vi "Format CSV.vi"(8 "error in (no error)":errorcluster, 9 "delimiter":string=",", 10 "CSV File Input":path, 11 "Original CSV Format":enum16{"OGnE", "WAN-OGE"}(ring)) -> (0 "error out":errorcluster, 1 "Parcel Length":i32[](array[numeric]), 3 "All Terminal Data":T1[](array[typedef]))   [LabVIEW 2017] (continued)
23:18:22.733", "2011-05-24 23:18:22.767", "2011-05-24 23:18:22.800", "2011-05-24 23:18:22.833", "2011-05-24 23:18:22.867", "2011-05-24 23:18:22.900", "2011-05-24 23:18:22.933", "2011-05-24 23:18:22.967", "2011-05-24 23:18:23.000", "2011-05-24 23:18:23.033", "2011-05-24 23:18:23.067", "2011-05-24 23:18:23.100", "2011-05-24 23:18:23.133", "2011-05-24 23:18:23.167", "2011-05-24 23:18:23.200", "2011-05-24 23:18:23.233", "2011-05-24 23:18:23.267", "2011-05-24 23:18:23.300", "2011-05-24 23:18:23.333", "2011-05-24 23:18:23.367", "2011-05-24 23:18:23.400", "2011-05-24 23:18:23.433", "2011-05-24 23:18:23.467", "2011-05-24 23:18:23.500", "2011-05-24 23:18:23.533", "2011-05-24 23:18:23.567", "2011-05-24 23:18:23.600", "2011-05-24 23:18:23.633", "2011-05-24 23:18:23.667", "2011-05-24 23:18:23.700", "2011-05-24 23:18:23.733", "2011-05-24 23:18:23.767", "2011-05-24 23:18:23.800", "2011-05-24 23:18:23.833", "2011-05-24 23:18:23.867", "2011-05-24 23:18:23.900", "2011-05-24 23:18:23.933", "2011-05-24 23:18:23.967", "2011-05-24 23:18:24.000", "2011-05-24 23:18:24.033", "2011-05-24 23:18:24.067", "2011-05-24 23:18:24.100", "2011-05-24 23:18:24.133", "2011-05-24 23:18:24.167", "2011-05-24 23:18:24.200", "2011-05-24 23:18:24.233", "2011-05-24 23:18:24.267", "2011-05-24 23:18:24.300", "2011-05-24 23:18:24.333", "2011-05-24 23:18:24.367", "2011-05-24 23:18:24.400", "2011-05-24 23:18:24.433", "2011-05-24 23:18:24.467", "2011-05-24 23:18:24.500", "2011-05-24 23:18:24.533", "2011-05-24 23:18:24.567", "2011-05-24 23:18:24.600", "2011-05-24 23:18:24.633", "2011-05-24 23:18:24.667", "2011-05-24 23:18:24.700", "2011-05-24 23:18:24.733", "2011-05-24 23:18:24.767", "2011-05-24 23:18:24.800", "2011-05-24 23:18:24.833", "2011-05-24 23:18:24.867", "2011-05-24 23:18:24.900", "2011-05-24 23:18:24.933", "2011-05-24 23:18:24.967", "2011-05-24 23:18:25.000", "2011-05-24 23:18:25.033", "2011-05-24 23:18:25.067", "2011-05-24 23:18:25.100", "2011-05-24 23:18:25.133", "2011-05-24 23:18:25.167", "2011-05-24 23:18:25.200", "2011-05-24 23:18:25.233", "2011-05-24 23:18:25.267", "2011-05-24 23:18:25.300", "2011-05-24 23:18:25.333", "2011-05-24 23:18:25.367", "2011-05-24 23:18:25.400", "2011-05-24 23:18:25.433", "2011-05-24 23:18:25.467", "2011-05-24 23:18:25.500", "2011-05-24 23:18:25.533", "2011-05-24 23:18:25.567", "2011-05-24 23:18:25.600", "2011-05-24 23:18:25.633", "2011-05-24 23:18:25.667", "2011-05-24 23:18:25.700", "2011-05-24 23:18:25.733", "2011-05-24 23:18:25.767", "2011-05-24 23:18:25.800", "2011-05-24 23:18:25.833", "2011-05-24 23:18:25.867", "2011-05-24 23:18:25.900", "2011-05-24 23:18:25.933", "2011-05-24 23:18:25.967", "2011-05-24 23:18:26.000", "2011-05-24 23:18:26.033", "2011-05-24 23:18:26.067", "2011-05-24 23:18:26.100", "2011-05-24 23:18:26.133", "2011-05-24 23:18:26.167", "2011-05-24 23:18:26.200", "2011-05-24 23:18:26.233", "2011-05-24 23:18:26.267", "2011-05-24 23:18:26.300", "2011-05-24 23:18:26.333", "2011-05-24 23:18:26.367", "2011-05-24 23:18:26.400", "2011-05-24 23:18:26.433", "2011-05-24 23:18:26.467", "2011-05-24 23:18:26.500", "2011-05-24 23:18:26.533", "2011-05-24 23:18:26.567", "2011-05-24 23:18:26.600", "2011-05-24 23:18:26.633", "2011-05-24 23:18:26.667", "2011-05-24 23:18:26.700", "2011-05-24 23:18:26.733", "2011-05-24 23:18:26.767", "2011-05-24 23:18:26.800", "2011-05-24 23:18:26.833", "2011-05-24 23:18:26.867", "2011-05-24 23:18:26.900", "2011-05-24 23:18:26.933", "2011-05-24 23:18:26.967", "2011-05-24 23:18:27.000", "2011-05-24 23:18:27.033", "2011-05-24 23:18:27.067", "2011-05-24 23:18:27.100", "2011-05-24 23:18:27.133", "2011-05-24 23:18:27.167", "2011-05-24 23:18:27.200", "2011-05-24 23:18:27.233", "2011-05-24 23:18:27.267", "2011-05-24 23:18:27.300", "2011-05-24 23:18:27.333", "2011-05-24 23:18:27.367", "2011-05-24 23:18:27.400", "2011-05-24 23:18:27.433", "2011-05-24 23:18:27.467", "2011-05-24 23:18:27.500", "2011-05-24 23:18:27.533", "2011-05-24 23:18:27.567", "2011-05-24 23:18:27.600", "2011-05-24 23:18:27.633", "2011-05-24 23:18:27.667", "2011-05-24 23:18:27.700", "2011-05-24 23:18:27.733", "2011-05-24 23:18:27.767", "2011-05-24 23:18:27.800", "2011-05-24 23:18:27.833", "2011-05-24 23:18:27.867", "2011-05-24 23:18:27.900", "2011-05-24 23:18:27.933", "2011-05-24 23:18:27.967", "2011-05-24 23:18:28.000", "2011-05-24 23:18:28.033", "2011-05-24 23:18:28.067", "2011-05-24 23:18:28.100", "2011-05-24 23:18:28.133", "2011-05-24 23:18:28.167", "2011-05-24 23:18:28.200", "2011-05-24 23:18:28.233", "2011-05-24 23:18:28.267", "2011-05-24 23:18:28.300", "2011-05-24 23:18:28.333", "2011-05-24 23:18:28.367", "2011-05-24 23:18:28.400", "2011-05-24 23:18:28.433", "2011-05-24 23:18:28.467", "2011-05-24 23:18:28.500", "2011-05-24 23:18:28.533", "2011-05-24 23:18:28.567", "2011-05-24 23:18:28.600", "2011-05-24 23:18:28.633", "2011-05-24 23:18:28.667", "2011-05-24 23:18:28.700", "2011-05-24 23:18:28.733", "2011-05-24 23:18:28.767", "2011-05-24 23:18:28.800", "2011-05-24 23:18:28.833", "2011-05-24 23:18:28.867", "2011-05-24 23:18:28.900", "2011-05-24 23:18:28.933", "2011-05-24 23:18:28.967", "2011-05-24 23:18:29.000", "2011-05-24 23:18:29.033", "2011-05-24 23:18:29.067", "2011-05-24 23:18:29.100", "2011-05-24 23:18:29.133", "2011-05-24 23:18:29.167", "2011-05-24 23:18:29.200", "2011-05-24 23:18:29.233", "2011-05-24 23:18:29.267", "2011-05-24 23:18:29.300", "2011-05-24 23:18:29.333", "2011-05-24 23:18:29.367", "2011-05-24 23:18:29.400", "2011-05-24 23:18:29.433", "2011-05-24 23:18:29.467", "2011-05-24 23:18:29.500", "2011-05-24 23:18:29.533", "2011-05-24 23:18:29.567", "2011-05-24 23:18:29.600", "2011-05-24 23:18:29.633", "2011-05-24 23:18:29.667", "2011-05-24 23:18:29.700", "2011-05-24 23:18:29.733", "2011-05-24 23:18:29.767", "2011-05-24 23:18:29.800", "2011-05-24 23:18:29.833", "2011-05-24 23:18:29.867", "2011-05-24 23:18:29.900", "2011-05-24 23:18:29.933", "2011-05-24 23:18:29.967", "2011-05-24 23:18:30.000", "2011-05-24 23:18:30.033", "2011-05-24 23:18:30.067", "2011-05-24 23:18:30.100", "2011-05-24 23:18:30.133", "2011-05-24 23:18:30.167", "2011-05-24 23:18:30.200", "2011-05-24 23:18:30.233", "2011-05-24 23:18:30.267", "2011-05-24 23:18:30.300", "2011-05-24 23:18:30.333", "2011-05-24 23:18:30.367", "2011-05-24 23:18:30.400", "2011-05-24 23:18:30.433", "2011-05-24 23:18:30.467", "2011-05-24 23:18:30.500", "2011-05-24 23:18:30.533", "2011-05-24 23:18:30.567", "2011-05-24 23:18:30.600", "2011-05-24 23:18:30.633", "2011-05-24 23:18:30.667", "2011-05-24 23:18:30.700", "2011-05-24 23:18:30.733", "2011-05-24 23:18:30.767", "2011-05-24 23:18:30.800", "2011-05-24 23:18:30.833", "2011-05-24 23:18:30.867", "2011-05-24 23:18:30.900", "2011-05-24 23:18:30.933", "2011-05-24 23:18:30.967", "2011-05-24 23:18:31.000", "2011-05-24 23:18:31.033", "2011-05-24 23:18:31.067", "2011-05-24 23:18:31.100", "2011-05-24 23:18:31.133", "2011-05-24 23:18:31.167", "2011-05-24 23:18:31.200", "2011-05-24 23:18:31.233", "2011-05-24 23:18:31.267", "2011-05-24 23:18:31.300", "2011-05-24 23:18:31.333", "2011-05-24 23:18:31.367", "2011-05-24 23:18:31.400", "2011-05-24 23:18:31.433", "2011-05-24 23:18:31.467", "2011-05-24 23:18:31.500", "2011-05-24 23:18:31.533", "2011-05-24 23:18:31.567", "2011-05-24 23:18:31.600", "2011-05-24 23:18:31.633", "2011-05-24 23:18:31.667", "2011-05-24 23:18:31.700", "2011-05-24 23:18:31.733", "2011-05-24 23:18:31.767", "2011-05-24 23:18:31.800", "2011-05-24 23:18:31.833", "2011-05-24 23:18:31.867", "2011-05-24 23:18:31.900", "2011-05-24 23:18:31.933", "2011-05-24 23:18:31.967", "2011-05-24 23:18:32.000", "2011-05-24 23:18:32.033", "2011-05-24 23:18:32.067", "2011-05-24 23:18:32.100", "2011-05-24 23:18:32.133", "2011-05-24 23:18:32.167", "2011-05-24 23:18:32.200", "2011-05-24 23:18:32.233", "2011-05-24 23:18:32.267", "2011-05-24 23:18:32.300", "2011-05-24 23:18:32.333", "2011-05-24 23:18:32.367", "2011-05-24 23:18:32.400", "2011-05-24 23:18:32.433", "2011-05-24 23:18:32.467", "2011-05-24 23:18:32.500", "2011-05-24 23:18:32.533", "2011-05-24 23:18:32.567", "2011-05-24 23:18:32.600", "2011-05-24 23:18:32.633", "2011-05-24 23:18:32.667", "2011-05-24 23:18:32.700", "2011-05-24 23:18:32.733", "2011-05-24 23:18:32.767", "2011-05-24 23:18:32.800", "2011-05-24 23:18:32.833", "2011-05-24 23:18:32.867", "2011-05-24 23:18:32.900", "2011-05-24 23:18:32.933", "2011-05-24 23:18:32.967", "2011-05-24 23:18:33.000", "2011-05-24 23:18:33.033", "2011-05-24 23:18:33.067", "2011-05-24 23:18:33.100", "2011-05-24 23:18:33.133", "2011-05-24 23:18:33.167", "2011-05-24 23:18:33.200", "2011-05-24 23:18:33.233", "2011-05-24 23:18:33.267", "2011-05-24 23:18:33.300", "2011-05-24 23:18:33.333", "2011-05-24 23:18:33.367", "2011-05-24 23:18:33.400", "2011-05-24 23:18:33.433", "2011-05-24 23:18:33.467", "2011-05-24 23:18:33.500", "2011-05-24 23:18:33.533", "2011-05-24 23:18:33.567", "2011-05-24 23:18:33.600", "2011-05-24 23:18:33.633", "2011-05-24 23:18:33.667", "2011-05-24 23:18:33.700", "2011-05-24 23:18:33.733", "2011-05-24 23:18:33.767", "2011-05-24 23:18:33.800", "2011-05-24 23:18:33.833", "2011-05-24 23:18:33.867", "2011-05-24 23:18:33.900", "2011-05-24 23:18:33.933", "2011-05-24 23:18:33.967", "2011-05-24 23:18:34.000", "2011-05-24 23:18:34.033", "2011-05-24 23:18:34.067", "2011-05-24 23:18:34.100", "2011-05-24 23:18:34.133", "2011-05-24 23:18:34.167", "2011-05-24 23:18:34.200", "2011-05-24 23:18:34.233", "2011-05-24 23:18:34.267", "2011-05-24 23:18:34.300", "2011-05-24 23:18:34.333", "2011-05-24 23:18:34.367", "2011-05-24 23:18:34.400", "2011-05-24 23:18:34.433", "2011-05-24 23:18:34.467", "2011-05-24 23:18:34.500", "2011-05-24 23:18:34.533", "2011-05-24 23:18:34.567", "2011-05-24 23:18:34.600", "2011-05-24 23:18:34.633", "2011-05-24 23:18:34.667", "2011-05-24 23:18:34.700", "2011-05-24 23:18:34.733", "2011-05-24 23:18:34.767", "2011-05-24 23:18:34.800", "2011-05-24 23:18:34.833", "2011-05-24 23:18:34.867", "2011-05-24 23:18:34.900", "2011-05-24 23:18:34.933", "2011-05-24 23:18:34.967", "2011-05-24 23:18:35.000", "2011-05-24 23:18:35.033", "2011-05-24 23:18:35.067", "2011-05-24 23:18:35.100", "2011-05-24 23:18:35.133", "2011-05-24 23:18:35.167", "2011-05-24 23:18:35.200", "2011-05-24 23:18:35.233", "2011-05-24 23:18:35.267", "2011-05-24 23:18:35.300", "2011-05-24 23:18:35.333", "2011-05-24 23:18:35.367", "2011-05-24 23:18:35.400", "2011-05-24 23:18:35.433", "2011-05-24 23:18:35.467", "2011-05-24 23:18:35.500", "2011-05-24 23:18:35.533", "2011-05-24 23:18:35.567", "2011-05-24 23:18:35.600", "2011-05-24 23:18:35.633", "2011-05-24 23:18:35.667", "2011-05-24 23:18:35.700", "2011-05-24 23:18:35.733", "2011-05-24 23:18:35.767", "2011-05-24 23:18:35.800", "2011-05-24 23:18:35.833", "2011-05-24 23:18:35.867", "2011-05-24 23:18:35.900", "2011-05-24 23:18:35.933", "2011-05-24 23:18:35.967", "2011-05-24 23:18:36.000", "2011-05-24 23:18:36.033", "2011-05-24 23:18:36.067", "2011-05-24 23:18:36.100", "2011-05-24 23:18:36.133", "2011-05-24 23:18:36.167", "2011-05-24 23:18:36.200", "2011-05-24 23:18:36.233", "2011-05-24 23:18:36.267", "2011-05-24 23:18:36.300", "2011-05-24 23:18:36.333", "2011-05-24 23:18:36.367", "2011-05-24 23:18:36.400", "2011-05-24 23:18:36.433", "2011-05-24 23:18:36.467", "2011-05-24 23:18:36.500", "2011-05-24 23:18:36.533", "2011-05-24 23:18:36.567", "2011-05-24 23:18:36.600", "2011-05-24 23:18:36.633", "2011-05-24 23:18:36.667", "2011-05-24 23:18:36.700", "2011-05-24 23:18:36.733", "2011-05-24 23:18:36.767", "2011-05-24 23:18:36.800", "2011-05-24 23:18:36.833", "2011-05-24 23:18:36.867", "2011-05-24 23:18:36.900", "2011-05-24 23:18:36.933", "2011-05-24 23:18:36.967", "2011-05-24 23:18:37.000", "2011-05-24 23:18:37.033", "2011-05-24 23:18:37.067", "2011-05-24 23:18:37.100", "2011-05-24 23:18:37.133", "2011-05-24 23:18:37.167", "2011-05-24 23:18:37.200", "2011-05-24 23:18:37.233", "2011-05-24 23:18:37.267", "2011-05-24 23:18:37.300", "2011-05-24 23:18:37.333", "2011-05-24 23:18:37.367", "2011-05-24 23:18:37.400", "2011-05-24 23:18:37.433", "2011-05-24 23:18:37.467", "2011-05-24 23:18:37.500", "2011-05-24 23:18:37.533", "2011-05-24 23:18:37.567", "2011-05-24 23:18:37.600", "2011-05-24 23:18:37.633", "2011-05-24 23:18:37.667", "2011-05-24 23:18:37.700", "2011-05-24 23:18:37.733", "2011-05-24 23:18:37.767", "2011-05-24 23:18:37.800", "2011-05-24 23:18:37.833", "2011-05-24 23:18:37.867", "2011-05-24 23:18:37.900", "2011-05-24 23:18:37.933", "2011-05-24 23:18:37.967", "2011-05-24 23:18:38.000", "2011-05-24 23:18:38.033", "2011-05-24 23:18:38.067", "2011-05-24 23:18:38.100", "2011-05-24 23:18:38.133", "2011-05-24 23:18:38.167", "2011-05-24 23:18:38.200", "2011-05-24 23:18:38.233", "2011-05-24 23:18:38.267", "2011-05-24 23:18:38.300", "2011-05-24 23:18:38.333", "2011-05-24 23:18:38.367", "2011-05-24 23:18:38.400", "2011-05-24 23:18:38.433", "2011-05-24 23:18:38.467", "2011-05-24 23:18:38.500", "2011-05-24 23:18:38.533", "2011-05-24 23:18:38.567", "2011-05-24 23:18:38.600", "2011-05-24 23:18:38.633", "2011-05-24 23:18:38.667", "2011-05-24 23:18:38.700", "2011-05-24 23:18:38.733", "2011-05-24 23:18:38.767", "2011-05-24 23:18:38.800", "2011-05-24 23:18:38.833", "2011-05-24 23:18:38.867", "2011-05-24 23:18:38.900", "2011-05-24 23:18:38.933", "2011-05-24 23:18:38.967", "2011-05-24 23:18:39.000", "2011-05-24 23:18:39.033", "2011-05-24 23:18:39.067", "2011-05-24 23:18:39.100", "2011-05-24 23:18:39.133", "2011-05-24 23:18:39.167", "2011-05-24 23:18:39.200", "2011-05-24 23:18:39.233", "2011-05-24 23:18:39.267", "2011-05-24 23:18:39.300", "2011-05-24 23:18:39.333", "2011-05-24 23:18:39.367", "2011-05-24 23:18:39.400", "2011-05-24 23:18:39.433", "2011-05-24 23:18:39.467", "2011-05-24 23:18:39.500", "2011-05-24 23:18:39.533", "2011-05-24 23:18:39.567", "2011-05-24 23:18:39.600", "2011-05-24 23:18:39.633", "2011-05-24 23:18:39.667", "2011-05-24 23:18:39.700", "2011-05-24 23:18:39.733", "2011-05-24 23:18:39.767", "2011-05-24 23:18:39.800", "2011-05-24 23:18:39.833", "2011-05-24 23:18:39.867", "2011-05-24 23:18:39.900", "2011-05-24 23:18:39.933", "2011-05-24 23:18:39.967", "2011-05-24 23:18:40.000", "2011-05-24 23:18:40.033", "2011-05-24 23:18:40.067", "2011-05-24 23:18:40.100", "2011-05-24 23:18:40.133", "2011-05-24 23:18:40.167", "2011-05-24 23:18:40.200", "2011-05-24 23:18:40.233", "2011-05-24 23:18:40.267", "2011-05-24 23:18:40.300", "2011-05-24 23:18:40.333", "2011-05-24 23:18:40.367", "2011-05-24 23:18:40.400", "2011-05-24 23:18:40.433", "2011-05-24 23:18:40.467", "2011-05-24 23:18:40.500", "2011-05-24 23:18:40.533", "2011-05-24 23:18:40.567", "2011-05-24 23:18:40.600", "2011-05-24 23:18:40.633", "2011-05-24 23:18:40.667", "2011-05-24 23:18:40.700", "2011-05-24 23:18:40.733", "2011-05-24 23:18:40.767", "2011-05-24 23:18:40.800", "2011-05-24 23:18:40.833", "2011-05-24 23:18:40.867", "2011-05-24 23:18:40.900", "2011-05-24 23:18:40.933", "2011-05-24 23:18:40.967", "2011-05-24 23:18:41.000", "2011-05-24 23:18:41.033", "2011-05-24 23:18:41.067", "2011-05-24 23:18:41.100", "2011-05-24 23:18:41.133", "2011-05-24 23:18:41.167", "2011-05-24 23:18:41.200", "2011-05-24 23:18:41.233", "2011-05-24 23:18:41.267", "2011-05-24 23:18:41.300", "2011-05-24 23:18:41.333", "2011-05-24 23:18:41.367", "2011-05-24 23:18:41.400", "2011-05-24 23:18:41.433", "2011-05-24 23:18:41.467", "2011-05-24 23:18:41.500", "2011-05-24 23:18:41.533", "2011-05-24 23:18:41.567", "2011-05-24 23:18:41.600", "2011-05-24 23:18:41.633", "2011-05-24 23:18:41.667", "2011-05-24 23:18:41.700", "2011-05-24 23:18:41.733", "2011-05-24 23:18:41.767", "2011-05-24 23:18:41.800", "2011-05-24 23:18:41.833", "2011-05-24 23:18:41.867", "2011-05-24 23:18:41.900", "2011-05-24 23:18:41.933", "2011-05-24 23:18:41.967", "2011-05-24 23:18:42.000", "2011-05-24 23:18:42.033", "2011-05-24 23:18:42.067", "2011-05-24 23:18:42.100", "2011-05-24 23:18:42.133", "2011-05-24 23:18:42.167", "2011-05-24 23:18:42.200", "2011-05-24 23:18:42.233", "2011-05-24 23:18:42.267", "2011-05-24 23:18:42.300", "2011-05-24 23:18:42.333", "2011-05-24 23:18:42.367", "2011-05-24 23:18:42.400", "2011-05-24 23:18:42.433", "2011-05-24 23:18:42.467", "2011-05-24 23:18:42.500", "2011-05-24 23:18:42.533", "2011-05-24 23:18:42.567", "2011-05-24 23:18:42.600", "2011-05-24 23:18:42.633", "2011-05-24 23:18:42.667", "2011-05-24 23:18:42.700", "2011-05-24 23:18:42.733", "2011-05-24 23:18:42.767", "2011-05-24 23:18:42.800", "2011-05-24 23:18:42.833", "2011-05-24 23:18:42.867", "2011-05-24 23:18:42.900", "2011-05-24 23:18:42.933", "2011-05-24 23:18:42.967", "2011-05-24 23:18:43.000", "2011-05-24 23:18:43.033", "2011-05-24 23:18:43.067", "2011-05-24 23:18:43.100", "2011-05-24 23:18:43.133", "2011-05-24 23:18:43.167", "2011-05-24 23:18:43.200", "2011-05-24 23:18:43.233", "2011-05-24 23:18:43.267", "2011-05-24 23:18:43.300", "2011-05-24 23:18:43.333", "2011-05-24 23:18:43.367", "2011-05-24 23:18:43.400", "2011-05-24 23:18:43.433", "2011-05-24 23:18:43.467", "2011-05-24 23:18:43.500", "2011-05-24 23:18:43.533", "2011-05-24 23:18:43.567", "2011-05-24 23:18:43.600", "2011-05-24 23:18:43.633", "2011-05-24 23:18:43.667", "2011-05-24 23:18:43.700", "2011-05-24 23:18:43.733", "2011-05-24 23:18:43.767", "2011-05-24 23:18:43.800", "2011-05-24 23:18:43.833", "2011-05-24 23:18:43.867", "2011-05-24 23:18:43.900", "2011-05-24 23:18:43.933", "2011-05-24 23:18:43.967", "2011-05-24 23:18:44.000", "2011-05-24 23:18:44.033", "2011-05-24 23:18:44.067", "2011-05-24 23:18:44.100", "2011-05-24 23:18:44.133", "2011-05-24 23:18:44.167", "2011-05-24 23:18:44.200", "2011-05-24 23:18:44.233", "2011-05-24 23:18:44.267", "2011-05-24 23:18:44.300", "2011-05-24 23:18:44.333", "2011-05-24 23:18:44.367", "2011-05-24 23:18:44.400", "2011-05-24 23:18:44.433", "2011-05-24 23:18:44.467", "2011-05-24 23:18:44.500", "2011-05-24 23:18:44.533", "2011-05-24 23:18:44.567", "2011-05-24 23:18:44.600", "2011-05-24 23:18:44.633", "2011-05-24 23:18:44.667", "2011-05-24 23:18:44.700", "2011-05-24 23:18:44.733", "2011-05-24 23:18:44.767", "2011-05-24 23:18:44.800", "2011-05-24 23:18:44.833", "2011-05-24 23:18:44.867", "2011-05-24 23:18:44.900", "2011-05-24 23:18:44.933", "2011-05-24 23:18:44.967", "2011-05-24 23:18:45.000", "2011-05-24 23:18:45.033", "2011-05-24 23:18:45.067", "2011-05-24 23:18:45.100", "2011-05-24 23:18:45.133", "2011-05-24 23:18:45.167", "2011-05-24 23:18:45.200", "2011-05-24 23:18:45.233", "2011-05-24 23:18:45.267", "2011-05-24 23:18:45.300", "2011-05-24 23:18:45.333", "2011-05-24 23:18:45.367", "2011-05-24 23:18:45.400", "2011-05-24 23:18:45.433", "2011-05-24 23:18:45.467", "2011-05-24 23:18:45.500", "2011-05-24 23:18:45.533", "2011-05-24 23:18:45.567", "2011-05-24 23:18:45.600", "2011-05-24 23:18:45.633", "2011-05-24 23:18:45.667", "2011-05-24 23:18:45.700", "2011-05-24 23:18:45.733", "2011-05-24 23:18:45.767", "2011-05-24 23:18:45.800", "2011-05-24 23:18:45.833", "2011-05-24 23:18:45.867", "2011-05-24 23:18:45.900", "2011-05-24 23:18:45.933", "2011-05-24 23:18:45.967", "2011-05-24 23:18:46.000", "2011-05-24 23:18:46.033", "2011-05-24 23:18:46.067", "2011-05-24 23:18:46.100", "2011-05-24 23:18:46.133", "2011-05-24 23:18:46.167", "2011-05-24 23:18:46.200", "2011-05-24 23:18:46.233", "2011-05-24 23:18:46.267", "2011-05-24 23:18:46.300", "2011-05-24 23:18:46.333", "2011-05-24 23:18:46.367", "2011-05-24 23:18:46.400", "2011-05-24 23:18:46.433", "2011-05-24 23:18:46.467", "2011-05-24 23:18:46.500", "2011-05-24 23:18:46.533", "2011-05-24 23:18:46.567", "2011-05-24 23:18:46.600", "2011-05-24 23:18:46.633", "2011-05-24 23:18:46.667", "2011-05-24 23:18:46.700", "2011-05-24 23:18:46.733", "2011-05-24 23:18:46.767", "2011-05-24 23:18:46.800", "2011-05-24 23:18:46.833", "2011-05-24 23:18:46.867", "2011-05-24 23:18:46.900", "2011-05-24 23:18:46.933", "2011-05-24 23:18:46.967", "2011-05-24 23:18:47.000", "2011-05-24 23:18:47.033", "2011-05-24 23:18:47.067", "2011-05-24 23:18:47.100", "2011-05-24 23:18:47.133", "2011-05-24 23:18:47.167", "2011-05-24 23:18:47.200", "2011-05-24 23:18:47.233", "2011-05-24 23:18:47.267", "2011-05-24 23:18:47.300", "2011-05-24 23:18:47.333", "2011-05-24 23:18:47.367", "2011-05-24 23:18:47.400", "2011-05-24 23:18:47.433", "2011-05-24 23:18:47.467", "2011-05-24 23:18:47.500", "2011-05-24 23:18:47.533", "2011-05-24 23:18:47.567", "2011-05-24 23:18:47.600", "2011-05-24 23:18:47.633", "2011-05-24 23:18:47.667", "2011-05-24 23:18:47.700", "2011-05-24 23:18:47.733", "2011-05-24 23:18:47.767", "2011-05-24 23:18:47.800", "2011-05-24 23:18:47.833", "2011-05-24 23:18:47.867", "2011-05-24 23:18:47.900", "2011-05-24 23:18:47.933", "2011-05-24 23:18:47.967", "2011-05-24 23:18:48.000", "2011-05-24 23:18:48.033", "2011-05-24 23:18:48.067", "2011-05-24 23:18:48.100", "2011-05-24 23:18:48.133", "2011-05-24 23:18:48.167", "2011-05-24 23:18:48.200", "2011-05-24 23:18:48.233", "2011-05-24 23:18:48.267", "2011-05-24 23:18:48.300", "2011-05-24 23:18:48.333", "2011-05-24 23:18:48.367", "2011-05-24 23:18:48.400", "2011-05-24 23:18:48.433", "2011-05-24 23:18:48.467", "2011-05-24 23:18:48.500", "2011-05-24 23:18:48.533", "2011-05-24 23:18:48.567", "2011-05-24 23:18:48.600", "2011-05-24 23:18:48.633", "2011-05-24 23:18:48.667", "2011-05-24 23:18:48.700", "2011-05-24 23:18:48.733", "2011-05-24 23:18:48.767", "2011-05-24 23:18:48.800", "2011-05-24 23:18:48.833", "2011-05-24 23:18:48.867", "2011-05-24 23:18:48.900", "2011-05-24 23:18:48.933", "2011-05-24 23:18:48.967", "2011-05-24 23:18:49.000", "2011-05-24 23:18:49.033", "2011-05-24 23:18:49.067", "2011-05-24 23:18:49.100", "2011-05-24 23:18:49.133", "2011-05-24 23:18:49.167", "2011-05-24 23:18:49.200", "2011-05-24 23:18:49.233", "2011-05-24 23:18:49.267", "2011-05-24 23:18:49.300", "2011-05-24 23:18:49.333", "2011-05-24 23:18:49.367", "2011-05-24 23:18:49.400", "2011-05-24 23:18:49.433", "2011-05-24 23:18:49.467", "2011-05-24 23:18:49.500", "2011-05-24 23:18:49.533", "2011-05-24 23:18:49.567", "2011-05-24 23:18:49.600", "2011-05-24 23:18:49.633", "2011-05-24 23:18:49.667", "2011-05-24 23:18:49.700", "2011-05-24 23:18:49.733", "2011-05-24 23:18:49.767", "2011-05-24 23:18:49.800", "2011-05-24 23:18:49.833", "2011-05-24 23:18:49.867", "2011-05-24 23:18:49.900", "2011-05-24 23:18:49.933", "2011-05-24 23:18:49.967", "2011-05-24 23:18:50.000", "2011-05-24 23:18:50.033", "2011-05-24 23:18:50.067", "2011-05-24 23:18:50.100", "2011-05-24 23:18:50.133", "2011-05-24 23:18:50.167", "2011-05-24 23:18:50.200", "2011-05-24 23:18:50.233", "2011-05-24 23:18:50.267", "2011-05-24 23:18:50.300", "2011-05-24 23:18:50.333", "2011-05-24 23:18:50.367", "2011-05-24 23:18:50.400", "2011-05-24 23:18:50.433", "2011-05-24 23:18:50.467", "2011-05-24 23:18:50.500", "2011-05-24 23:18:50.533", "2011-05-24 23:18:50.567", "2011-05-24 23:18:50.600", "2011-05-24 23:18:50.633", "2011-05-24 23:18:50.667", "2011-05-24 23:18:50.700", "2011-05-24 23:18:50.733", "2011-05-24 23:18:50.767", "2011-05-24 23:18:50.800", "2011-05-24 23:18:50.833", "2011-05-24 23:18:50.867", "2011-05-24 23:18:50.900", "2011-05-24 23:18:50.933", "2011-05-24 23:18:50.967", "2011-05-24 23:18:51.000", "2011-05-24 23:18:51.033", "2011-05-24 23:18:51.067", "2011-05-24 23:18:51.100", "2011-05-24 23:18:51.133", "2011-05-24 23:18:51.167", "2011-05-24 23:18:51.200", "2011-05-24 23:18:51.233", "2011-05-24 23:18:51.267", "2011-05-24 23:18:51.300", "2011-05-24 23:18:51.333", "2011-05-24 23:18:51.367", "2011-05-24 23:18:51.400", "2011-05-24 23:18:51.433", "2011-05-24 23:18:51.467", "2011-05-24 23:18:51.500", "2011-05-24 23:18:51.533", "2011-05-24 23:18:51.567", "2011-05-24 23:18:51.600", "2011-05-24 23:18:51.633", "2011-05-24 23:18:51.667", "2011-05-24 23:18:51.700", "2011-05-24 23:18:51.733", "2011-05-24 23:18:51.767", "2011-05-24 23:18:51.800", "2011-05-24 23:18:51.833", "2011-05-24 23:18:51.867", "2011-05-24 23:18:51.900", "2011-05-24 23:18:51.933", "2011-05-24 23:18:51.967", "2011-05-24 23:18:52.000", "2011-05-24 23:18:52.033", "2011-05-24 23:18:52.067", "2011-05-24 23:18:52.100", "2011-05-24 23:18:52.133", "2011-05-24 23:18:52.167", "2011-05-24 23:18:52.200", "2011-05-24 23:18:52.233", "2011-05-24 23:18:52.267", "2011-05-24 23:18:52.300", "2011-05-24 23:18:52.333", "2011-05-24 23:18:52.367", "2011-05-24 23:18:52.400", "2011-05-24 23:18:52.433", "2011-05-24 23:18:52.467", "2011-05-24 23:18:52.500", "2011-05-24 23:18:52.533", "2011-05-24 23:18:52.567", "2011-05-24 23:18:52.600", "2011-05-24 23:18:52.633", "2011-05-24 23:18:52.667", "2011-05-24 23:18:52.700", "2011-05-24 23:18:52.733", "2011-05-24 23:18:52.767", "2011-05-24 23:18:52.800", "2011-05-24 23:18:52.833", "2011-05-24 23:18:52.867", "2011-05-24 23:18:52.900", "2011-05-24 23:18:52.933", "2011-05-24 23:18:52.967", "2011-05-24 23:18:53.000", "2011-05-24 23:18:53.033", "2011-05-24 23:18:53.067", "2011-05-24 23:18:53.100", "2011-05-24 23:18:53.133", "2011-05-24 23:18:53.167", "2011-05-24 23:18:53.200", "2011-05-24 23:18:53.233", "2011-05-24 23:18:53.267", "2011-05-24 23:18:53.300", "2011-05-24 23:18:53.333", "2011-05-24 23:18:53.367", "2011-05-24 23:18:53.400", "2011-05-24 23:18:53.433", "2011-05-24 23:18:53.467", "2011-05-24 23:18:53.500", "2011-05-24 23:18:53.533", "2011-05-24 23:18:53.567", "2011-05-24 23:18:53.600", "2011-05-24 23:18:53.633", "2011-05-24 23:18:53.667", "2011-05-24 23:18:53.700", "2011-05-24 23:18:53.733", "2011-05-24 23:18:53.767", "2011-05-24 23:18:53.800", "2011-05-24 23:18:53.833", "2011-05-24 23:18:53.867", "2011-05-24 23:18:53.900", "2011-05-24 23:18:53.933", "2011-05-24 23:18:53.967", "2011-05-24 23:18:54.000", "2011-05-24 23:18:54.033", "2011-05-24 23:18:54.067", "2011-05-24 23:18:54.100", "2011-05-24 23:18:54.133", "2011-05-24 23:18:54.167", "2011-05-24 23:18:54.200", "2011-05-24 23:18:54.233", "2011-05-24 23:18:54.267", "2011-05-24 23:18:54.300", "2011-05-24 23:18:54.333", "2011-05-24 23:18:54.367", "2011-05-24 23:18:54.400", "2011-05-24 23:18:54.433", "2011-05-24 23:18:54.467", "2011-05-24 23:18:54.500", "2011-05-24 23:18:54.533", "2011-05-24 23:18:54.567", "2011-05-24 23:18:54.600", "2011-05-24 23:18:54.633", "2011-05-24 23:18:54.667", "2011-05-24 23:18:54.700", "2011-05-24 23:18:54.733", "2011-05-24 23:18:54.767", "2011-05-24 23:18:54.800", "2011-05-24 23:18:54.833", "2011-05-24 23:18:54.867", "2011-05-24 23:18:54.900", "2011-05-24 23:18:54.933", "2011-05-24 23:18:54.967", "2011-05-24 23:18:55.000", "2011-05-24 23:18:55.033", "2011-05-24 23:18:55.067", "2011-05-24 23:18:55.100", "2011-05-24 23:18:55.133", "2011-05-24 23:18:55.167", "2011-05-24 23:18:55.200", "2011-05-24 23:18:55.233", "2011-05-24 23:18:55.267", "2011-05-24 23:18:55.300", "2011-05-24 23:18:55.333", "2011-05-24 23:18:55.367", "2011-05-24 23:18:55.400", "2011-05-24 23:18:55.433", "2011-05-24 23:18:55.467", "2011-05-24 23:18:55.500", "2011-05-24 23:18:55.533", "2011-05-24 23:18:55.567", "2011-05-24 23:18:55.600", "2011-05-24 23:18:55.633", "2011-05-24 23:18:55.667", "2011-05-24 23:18:55.700", "2011-05-24 23:18:55.733", "2011-05-24 23:18:55.767", "2011-05-24 23:18:55.800", "2011-05-24 23:18:55.833", "2011-05-24 23:18:55.867", "2011-05-24 23:18:55.900", "2011-05-24 23:18:55.933", "2011-05-24 23:18:55.967", "2011-05-24 23:18:56.000", "2011-05-24 23:18:56.033", "2011-05-24 23:18:56.067", "2011-05-24 23:18:56.100", "2011-05-24 23:18:56.133", "2011-05-24 23:18:56.167", "2011-05-24 23:18:56.200", "2011-05-24 23:18:56.233", "2011-05-24 23:18:56.267", "2011-05-24 23:18:56.300", "2011-05-24 23:18:56.333", "2011-05-24 23:18:56.367", "2011-05-24 23:18:56.400", "2011-05-24 23:18:56.433", "2011-05-24 23:18:56.467", "2011-05-24 23:18:56.500", "2011-05-24 23:18:56.533", "2011-05-24 23:18:56.567", "2011-05-24 23:18:56.600", "2011-05-24 23:18:56.633", "2011-05-24 23:18:56.667", "2011-05-24 23:18:56.700", "2011-05-24 23:18:56.733", "2011-05-24 23:18:56.767", "2011-05-24 23:18:56.800", "2011-05-24 23:18:56.833", "2011-05-24 23:18:56.867", "2011-05-24 23:18:56.900", "2011-05-24 23:18:56.933", "2011-05-24 23:18:56.967", "2011-05-24 23:18:57.000", "2011-05-24 23:18:57.033", "2011-05-24 23:18:57.067", "2011-05-24 23:18:57.100", "2011-05-24 23:18:57.133", "2011-05-24 23:18:57.167", "2011-05-24 23:18:57.200", "2011-05-24 23:18:57.233", "2011-05-24 23:18:57.267", "2011-05-24 23:18:57.300", "2011-05-24 23:18:57.333", "2011-05-24 23:18:57.367", "2011-05-24 23:18:57.400", "2011-05-24 23:18:57.433", "2011-05-24 23:18:57.467", "2011-05-24 23:18:57.500", "2011-05-24 23:18:57.533", "2011-05-24 23:18:57.567", "2011-05-24 23:18:57.600", "2011-05-24 23:18:57.633", "2011-05-24 23:18:57.667", "2011-05-24 23:18:57.700", "2011-05-24 23:18:57.733", "2011-05-24 23:18:57.767", "2011-05-24 23:18:57.800", "2011-05-24 23:18:57.833", "2011-05-24 23:18:57.867", "2011-05-24 23:18:57.900", "2011-05-24 23:18:57.933", "2011-05-24 23:18:57.967", "2011-05-24 23:18:58.000", "2011-05-24 23:18:58.033", "2011-05-24 23:18:58.067", "2011-05-24 23:18:58.100", "2011-05-24 23:18:58.133", "2011-05-24 23:18:58.167", "2011-05-24 23:18:58.200", "2011-05-24 23:18:58.233", "2011-05-24 23:18:58.267", "2011-05-24 23:18:58.300", "2011-05-24 23:18:58.333", "2011-05-24 23:18:58.367", "2011-05-24 23:18:58.400", "2011-05-24 23:18:58.433", "2011-05-24 23:18:58.467", "2011-05-24 23:18:58.500", "2011-05-24 23:18:58.533", "2011-05-24 23:18:58.567", "2011-05-24 23:18:58.600", "2011-05-24 23:18:58.633", "2011-05-24 23:18:58.667", "2011-05-24 23:18:58.700", "2011-05-24 23:18:58.733", "2011-05-24 23:18:58.767", "2011-05-24 23:18:58.800", "2011-05-24 23:18:58.833", "2011-05-24 23:18:58.867", "2011-05-24 23:18:58.900", "2011-05-24 23:18:58.933", "2011-05-24 23:18:58.967", "2011-05-24 23:18:59.000", "2011-05-24 23:18:59.033", "2011-05-24 23:18:59.067", "2011-05-24 23:18:59.100", "2011-05-24 23:18:59.133", "2011-05-24 23:18:59.167", "2011-05-24 23:18:59.200", "2011-05-24 23:18:59.233", "2011-05-24 23:18:59.267", "2011-05-24 23:18:59.300", "2011-05-24 23:18:59.333", "2011-05-24 23:18:59.367", "2011-05-24 23:18:59.400", "2011-05-24 23:18:59.433", "2011-05-24 23:18:59.467", "2011-05-24 23:18:59.500", "2011-05-24 23:18:59.533", "2011-05-24 23:18:59.567", "2011-05-24 23:18:59.600", "2011-05-24 23:18:59.633", "2011-05-24 23:18:59.667", "2011-05-24 23:18:59.700", "2011-05-24 23:18:59.733", "2011-05-24 23:18:59.767", "2011-05-24 23:18:59.800", "2011-05-24 23:18:59.833", "2011-05-24 23:18:59.867", "2011-05-24 23:18:59.900", "2011-05-24 23:18:59.933", "2011-05-24 23:18:59.967", "2011-05-24 23:19:00.000", "2011-05-24 23:19:00.033", "2011-05-24 23:19:00.067", "2011-05-24 23:19:00.100", "2011-05-24 23:19:00.133", "2011-05-24 23:19:00.167", "2011-05-24 23:19:00.200", "2011-05-24 23:19:00.233", "2011-05-24 23:19:00.267", "2011-05-24 23:19:00.300", "2011-05-24 23:19:00.333", "2011-05-24 23:19:00.367", "2011-05-24 23:19:00.400", "2011-05-24 23:19:00.433", "2011-05-24 23:19:00.467", "2011-05-24 23:19:00.500", "2011-05-24 23:19:00.533", "2011-05-24 23:19:00.567", "2011-05-24 23:19:00.600", "2011-05-24 23:19:00.633", "2011-05-24 23:19:00.667", "2011-05-24 23:19:00.700", "2011-05-24 23:19:00.733", "2011-05-24 23:19:00.767", "2011-05-24 23:19:00.800", "2011-05-24 23:19:00.833", "2011-05-24 23:19:00.867", "2011-05-24 23:19:00.900", "2011-05-24 23:19:00.933", "2011-05-24 23:19:00.967", "2011-05-24 23:19:01.000", "2011-05-24 23:19:01.033", "2011-05-24 23:19:01.067", "2011-05-24 23:19:01.100", "2011-05-24 23:19:01.133", "2011-05-24 23:19:01.167", "2011-05-24 23:19:01.200", "2011-05-24 23:19:01.233", "2011-05-24 23:19:01.267", "2011-05-24 23:19:01.300", "2011-05-24 23:19:01.333", "2011-05-24 23:19:01.367", "2011-05-24 23:19:01.400", "2011-05-24 23:19:01.433", "2011-05-24 23:19:01.467", "2011-05-24 23:19:01.500", "2011-05-24 23:19:01.533", "2011-05-24 23:19:01.567", "2011-05-24 23:19:01.600", "2011-05-24 23:19:01.633", "2011-05-24 23:19:01.667", "2011-05-24 23:19:01.700", "2011-05-24 23:19:01.733", "2011-05-24 23:19:01.767", "2011-05-24 23:19:01.800", "2011-05-24 23:19:01.833", "2011-05-24 23:19:01.867", "2011-05-24 23:19:01.900", "2011-05-24 23:19:01.933", "2011-05-24 23:19:01.967", "2011-05-24 23:19:02.000", "2011-05-24 23:19:02.033", "2011-05-24 23:19:02.067", "2011-05-24 23:19:02.100", "2011-05-24 23:19:02.133", "2011-05-24 23:19:02.167", "2011-05-24 23:19:02.200", "2011-05-24 23:19:02.233", "2011-05-24 23:19:02.267", "2011-05-24 23:19:02.300", "2011-05-24 23:19:02.333", "2011-05-24 23:19:02.367", "2011-05-24 23:19:02.400", "2011-05-24 23:19:02.433", "2011-05-24 23:19:02.467", "2011-05-24 23:19:02.500", "2011-05-24 23:19:02.533", "2011-05-24 23:19:02.567", "2011-05-24 23:19:02.600", "2011-05-24 23:19:02.633", "2011-05-24 23:19:02.667", "2011-05-24 23:19:02.700", "2011-05-24 23:19:02.733", "2011-05-24 23:19:02.767", "2011-05-24 23:19:02.800", "2011-05-24 23:19:02.833", "2011-05-24 23:19:02.867", "2011-05-24 23:19:02.900", "2011-05-24 23:19:02.933", "2011-05-24 23:19:02.967", "2011-05-24 23:19:03.000", "2011-05-24 23:19:03.033", "2011-05-24 23:19:03.067", "2011-05-24 23:19:03.100", "2011-05-24 23:19:03.133", "2011-05-24 23:19:03.167", "2011-05-24 23:19:03.200", "2011-05-24 23:19:03.233", "2011-05-24 23:19:03.267", "2011-05-24 23:19:03.300", "2011-05-24 23:19:03.333", "2011-05-24 23:19:03.367", "2011-05-24 23:19:03.400", "2011-05-24 23:19:03.433", "2011-05-24 23:19:03.467", "2011-05-24 23:19:03.500", "2011-05-24 23:19:03.533", "2011-05-24 23:19:03.567", "2011-05-24 23:19:03.600", "2011-05-24 23:19:03.633", "2011-05-24 23:19:03.667", "2011-05-24 23:19:03.700", "2011-05-24 23:19:03.733", "2011-05-24 23:19:03.767", "2011-05-24 23:19:03.800", "2011-05-24 23:19:03.833", "2011-05-24 23:19:03.867", "2011-05-24 23:19:03.900", "2011-05-24 23:19:03.933", "2011-05-24 23:19:03.967", "2011-05-24 23:19:04.000", "2011-05-24 23:19:04.033", "2011-05-24 23:19:04.067", "2011-05-24 23:19:04.100", "2011-05-24 23:19:04.133", "2011-05-24 23:19:04.167", "2011-05-24 23:19:04.200", "2011-05-24 23:19:04.233", "2011-05-24 23:19:04.267", "2011-05-24 23:19:04.300", "2011-05-24 23:19:04.333", "2011-05-24 23:19:04.367", "2011-05-24 23:19:04.400", "2011-05-24 23:19:04.433", "2011-05-24 23:19:04.467", "2011-05-24 23:19:04.500", "2011-05-24 23:19:04.533", "2011-05-24 23:19:04.567", "2011-05-24 23:19:04.600", "2011-05-24 23:19:04.633", "2011-05-24 23:19:04.667", "2011-05-24 23:19:04.700", "2011-05-24 23:19:04.733", "2011-05-24 23:19:04.767", "2011-05-24 23:19:04.800", "2011-05-24 23:19:04.833", "2011-05-24 23:19:04.867", "2011-05-24 23:19:04.900", "2011-05-24 23:19:04.933", "2011-05-24 23:19:04.967", "2011-05-24 23:19:05.000", "2011-05-24 23:19:05.033", "2011-05-24 23:19:05.067", "2011-05-24 23:19:05.100", "2011-05-24 23:19:05.133", "2011-05-24 23:19:05.167", "2011-05-24 23:19:05.200", "2011-05-24 23:19:05.233", "2011-05-24 23:19:05.267", "2011-05-24 23:19:05.300", "2011-05-24 23:19:05.333", "2011-05-24 23:19:05.367", "2011-05-24 23:19:05.400", "2011-05-24 23:19:05.433", "2011-05-24 23:19:05.467", "2011-05-24 23:19:05.500", "2011-05-24 23:19:05.533", "2011-05-24 23:19:05.567", "2011-05-24 23:19:05.600", "2011-05-24 23:19:05.633", "2011-05-24 23:19:05.667", "2011-05-24 23:19:05.700", "2011-05-24 23:19:05.733", "2011-05-24 23:19:05.767", "2011-05-24 23:19:05.800", "2011-05-24 23:19:05.833", "2011-05-24 23:19:05.867", "2011-05-24 23:19:05.900"]
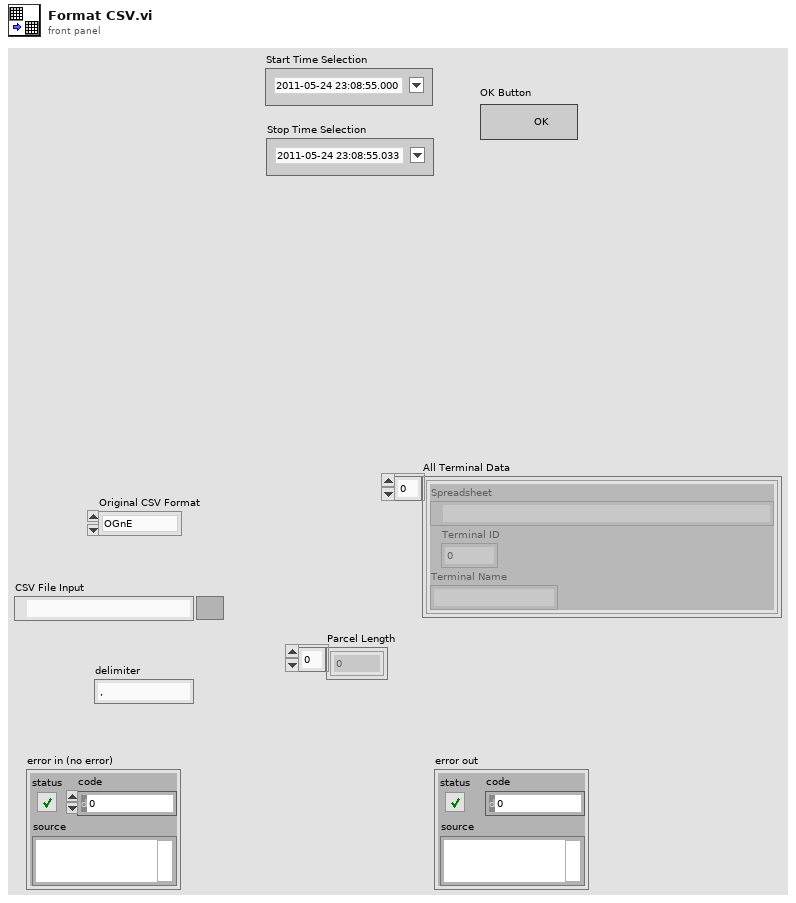
[diagram p1: front panel]
types:
  T1 = typedef "Terminal Data.ctl" = cluster{"Spreadsheet":path, "Terminal ID":u32, "Terminal Name":string}
  T2 = enum8{"Enabled", "Disabled", "Disabled and Grayed Out"}
  T3 = cluster{"Terminal Data":path, "Terminal ID":dbl, "Terminal Name":string}
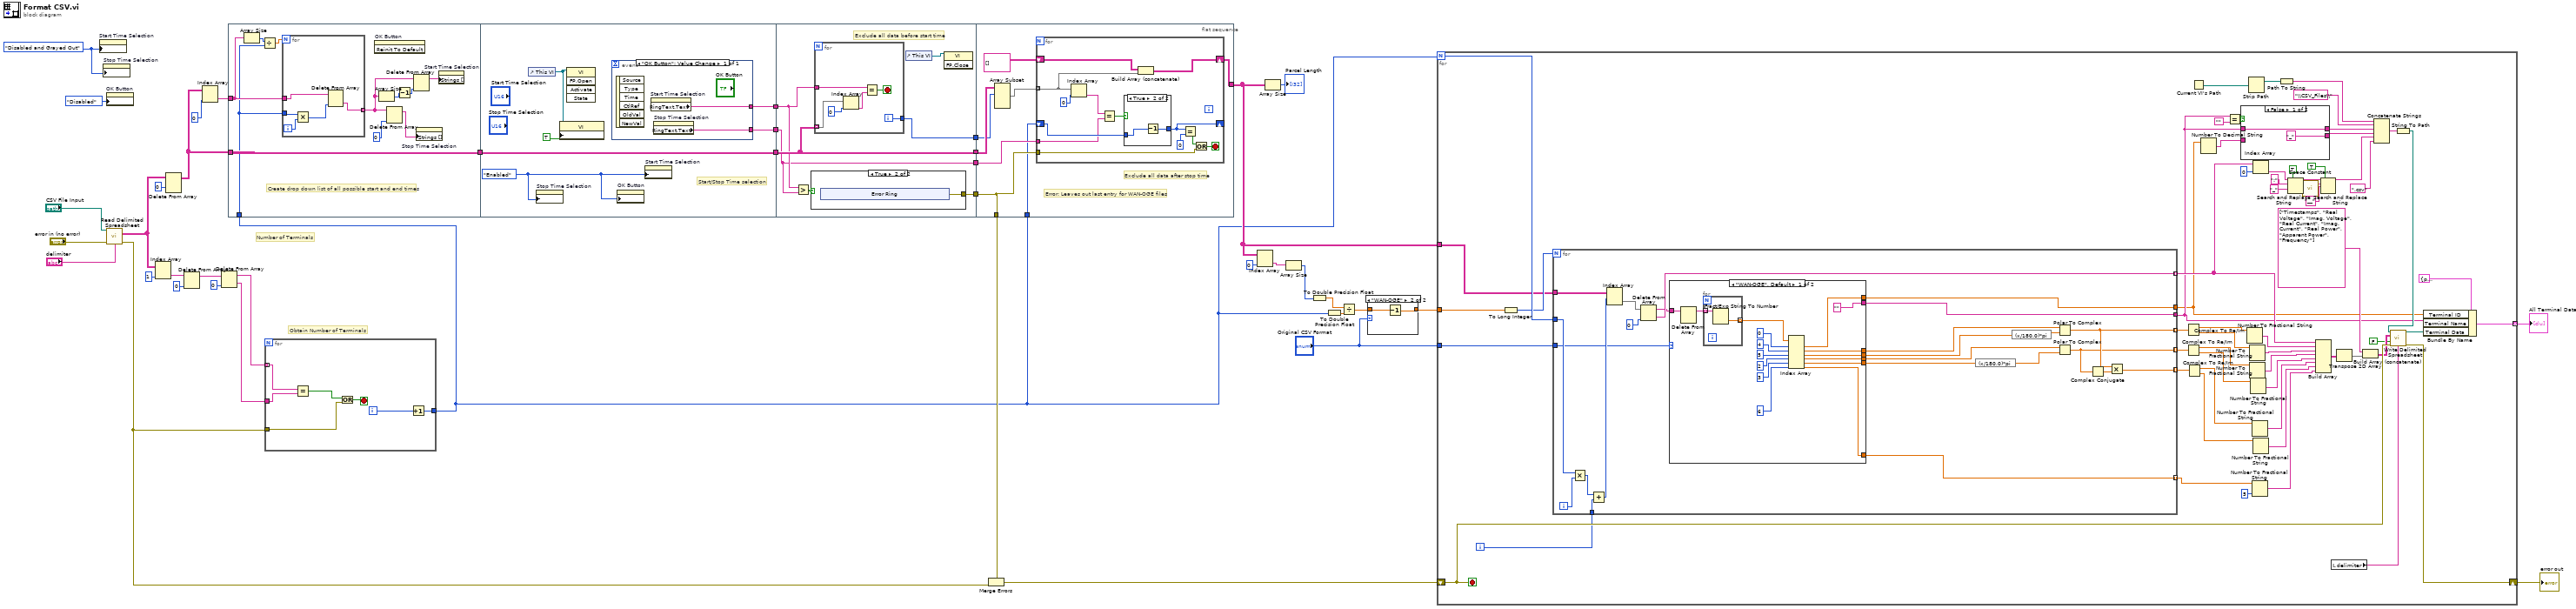
[diagram p0: block diagram]
diagram:
  w2 = T2."Disabled and Grayed Out" ("Disabled")
  # "Obtain Number of Terminals"
  # "Number of Terminals"
  n1 = property on="Start Time Selection" class="Ring (strict)"("DisabledEnum"=w2) -> ()  [unwired: 2 in, 2 out]
  n2 = property on="Stop Time Selection" class="Ring (strict)"("DisabledEnum"=w2) -> ()  [unwired: 2 in, 2 out]
  n3 = property on="OK Button" class="Bool"("DisabledEnum"=T2."Disabled" ("Disabled")) -> ()  [unwired: 2 in, 2 out]
  n4 = call-poly <vilib>:"Read Delimited Spreadsheet.vi"("file path (dialog if empty)"="CSV File Input", "error in (no error)"="error in (no error)", "delimiter (\\t)"="delimiter") -> ("all rows"=w21:string[][], "error out"=w12:errorcluster)  [unwired: 7 in, 4 out]
  n5 = Index Array(array=w21, index (col)=1 ("disabled index (col)")) -> (element=w27:string[])  [unwired: 1 in]
  n6 = Delete From Array(array=w21, index (row)=0) -> (array with subset deleted=w19:string[][])  [unwired: 2 in, 1 out]
  n7 = Delete From Array(array=w27, index=0) -> (array with subset deleted=w26:string[])  [unwired: 1 in, 1 out]
  n8 = Index Array(array=w19, index (col)=0 ("disabled index (col)")) -> (element=w22:string[])  [unwired: 1 in]
  n9 = Delete From Array(array=w26, index=0) -> (deleted portion=w35:string, array with subset deleted=w36:string[])  [unwired: 1 in]
  n10 = flat-sequence {
    tunnel: [w52] -> w24
    tunnel: w19 -> [w52]
    tunnel: w22 -> [w51]
    tunnel: w3 -> [w46]
    tunnel: w24 -> [w63]
    tunnel: [w63] -> w18
    tunnel: [w60] -> w17
    tunnel: [w59] -> w16
    tunnel: w18 -> [w72]
    tunnel: w17 -> [w70]
    tunnel: w16 -> [w69]
    tunnel: [w69] -> w15
    tunnel: [w72] -> w14
    tunnel: [w71] -> w13
    tunnel: [w67] -> w10
    tunnel: [w94] -> w5
    tunnel: w15 -> [w91]
    tunnel: w14 -> [w92]
    tunnel: w13 -> [w90]
    tunnel: w3 -> [w87]
    tunnel: w10 -> [w88]
    tunnel: [w88] -> w9
    frame #0 {
      # "Create drop down list of all possible start and end times"
      n11 = Array Size(array=w51) -> (size(s)=w50:i32)
      n12 = Divide(x=w50, y=w46) -> (x/y=w49:dbl)
      n13 = for {
        N: w49 -> [_]
        tunnel: w51 -> [w55]
        tunnel: [w53] -> w45 mode=indexing
        tunnel: w46 -> [w56]
        i -> [w57]
        n14 = Multiply(x=w56, y=w57) -> (x*y=w54:i32)
        n15 = Delete From Array(array=w55, index=w54) -> (deleted portion=w53:string)  [unwired: 1 in, 1 out]
      }
      n16 = invoke on="OK Button" class="Bool" method="Reinit To Default"() -> ()  [unwired: 3 in, 3 out]
      n17 = Array Size(array=w45) -> (size(s)=w44:i32)
      n18 = Delete From Array(array=w45, index=0) -> (array with subset deleted=w47:string[])  [unwired: 1 in, 1 out]
      n19 = Decrement(x=w44) -> (x-1=w43:i32)
      n20 = Delete From Array(array=w45, index=w43) -> (array with subset deleted=w42:string[])  [unwired: 1 in, 1 out]
      n21 = property on="Stop Time Selection" class="Ring (strict)"("Strings []"=w47) -> ()  [unwired: 2 in, 2 out]
      n22 = property on="Start Time Selection" class="Ring (strict)"("Strings []"=w42) -> ()  [unwired: 2 in, 2 out]
    }
    frame #1 {
      w58 = T2."Enabled" ("Disabled")
      # "Start/Stop Time selection"
      n23 = control-ref of="This VI"() -> (w62:refnum<vi>)
      n24 = property on="Stop Time Selection" class="Ring (strict)"("DisabledEnum"=w58) -> ()  [unwired: 2 in, 2 out]
      n25 = property class="VI"(reference=w62, "Front Panel.IsFrontmost"=TRUE ("Front Panel Window:Is Frontmost")) -> ()  [unwired: 1 in, 2 out]
      n26 = invoke class="VI" method="FP.Open"(reference=w62) -> ()  [unwired: 4 in, 5 out]
      n27 = event shown="[0] \"OK Button\": Value Change" {
        selector: _ -> [_]
        dyn-events: _ -> [_]
        timeout: _ -> [_]
        tunnel: [w65] -> w60
        tunnel: [w64] -> w59
        event "OK Button": Value Change {
          n28 = event-data() -> ()  [unwired: 1 in, 6 out]
          n29 = property on="Start Time Selection" class="Ring (strict)"() -> ("RingText.Text"=w65:string)  [unwired: 2 in, 2 out]
          n30 = property on="Stop Time Selection" class="Ring (strict)"() -> ("RingText.Text"=w64:string)  [unwired: 2 in, 2 out]
        }
      }
      n31 = property on="OK Button" class="Bool"("DisabledEnum"=w58) -> ()  [unwired: 2 in, 2 out]
      n32 = property on="Start Time Selection" class="Ring (strict)"("DisabledEnum"=w58) -> ()  [unwired: 2 in, 2 out]
    }
    frame #2 {
      # "Exclude all data before start time"
      n33 = Greater?(x=w70, y=w69) -> (0:w68:bool)
      n34 = case shown="True" w68 {
        tunnel: [w73 w75] -> w67
        frame False {
          n35 = xnode "Error Ring"() -> ("error out"=w73:errorcluster)
        }
        frame True {
          n36 = xnode "Error Ring"() -> ("error out"=w75:errorcluster)
        }
      }
      n37 = for {
        tunnel: w72 -> [w85] mode=indexing
        tunnel: w70 -> [w83]
        tunnel: [w81] -> w71
        i -> [w81]
        stop <- w82 stop-if-true
        n38 = Index Array(array=w85, index=0) -> (element=w84:string)
        n39 = Equal?(x=w83, y=w84) -> (x = y?=w82:bool)
      }
      n40 = control-ref of="This VI"() -> (w66:refnum<vi>)
      n41 = invoke class="VI" method="FP.Close"(reference=w66) -> ()  [unwired: 2 in, 3 out]
    }
    frame #3 {
      # "Error: Leaves out last entry for WAN-OGE files"
      # "Exclude all data after stop time"
      n42 = Array Subset(array=w92, index (row)=w90) -> (w89:string[][])  [unwired: 3 in]
      n43 = for {
        shift-right: [w106] -> w94
        shift-left: string[][] [] ("all rows") -> [w107]
        tunnel: w91 -> [w96]
        tunnel: w89 -> [w103] mode=indexing
        tunnel: w88 -> [w97]
        shift-right: [w95] -> _
        shift-left: w87 -> [w100]
        stop <- w98 stop-if-true
        n44 = Index Array "Index Array"(array=w103, index=0) -> (element=w104:string)
        n45 = Equal?(x=w104, y=w96) -> (x = y?=w102:bool)
        n46 = case shown="True" w102 {
          tunnel: w100 -> [w108 w110]
          tunnel: [w108 w109] -> w95
          frame False {
          }
          frame True {
            n47 = Decrement(x=w110) -> (x-1=w109:i32)
          }
        }
        n48 = Build Array (concatenate)(w107, w103) -> (w106:string[][])
        n49 = Equal?(x=w95, y=0 ("index")) -> (x = y?=w99:bool)
        n50 = Or(x=w99, y=w97) -> (x .or. y?=w98:bool)
      }
    }
  }
  n51 = for {
    tunnel: w36 -> [w115] mode=indexing
    tunnel: w35 -> [w114]
    tunnel: [w116] -> w3
    tunnel: w12 -> [w113]
    i -> [w117]
    stop <- w111 stop-if-true
    n52 = Equal?(x=w115, y=w114) -> (x = y?=w112:bool)
    n53 = Or(x=w112, y=w113) -> (x .or. y?=w111:bool)
    n54 = Increment(x=w117) -> (x+1=w116:i32)
  }
  n55 = Merge Errors(w9, w12) -> (w11:errorcluster)
  n56 = Index Array(array=w5, index (col)=0 ("disabled index (col)")) -> (element=w32:string[])  [unwired: 1 in]
  n57 = Array Size(array=w5) -> (size(s)=→"Parcel Length":i32[])
  n58 = Array Size(array=w32) -> (size(s)=w31:i32)
  n59 = To Double Precision Float(number=w31) -> (double precision float=w29:dbl)
  n60 = To Double Precision Float(number=w3) -> (double precision float=w30:dbl)
  n61 = Divide(x=w29, y=w30) -> (x/y=w7:dbl)
  n62 = case shown="\"WAN-OGE\"" "Original CSV Format" {
    tunnel: w7 -> [w118 w120]
    tunnel: [w118 w119] -> w6
    frame "OGnE" {
    }
    frame "WAN-OGE" {
      n63 = Decrement(x=w120) -> (x-1=w119:dbl)
    }
  }
  n64 = for {
    N: w3 -> [w178]
    shift-right: [w179] -> w41
    shift-left: w11 -> [w180]
    tunnel: w5 -> [w126]
    tunnel: "Original CSV Format" -> [w128]
    tunnel: w6 -> [w127]
    tunnel: [w173] -> w28 mode=indexing
    i -> [w177]
    stop <- w180 stop-if-true
    n65 = To Long Integer(number=w127) -> (32bit integer=w176:i32)
    n66 = for {
      N: w176 -> [_]
      tunnel: w126 -> [w190]
      tunnel: w128 -> [w204]
      tunnel: w178 -> [w210]
      tunnel: w177 -> [w208]
      tunnel: [w195] -> w171 mode=indexing
      tunnel: [w194] -> w170 mode=indexing
      tunnel: [w192] -> w169 mode=indexing
      tunnel: [w203] -> w132
      tunnel: [w188] -> w151 mode=indexing
      tunnel: [w202] -> w130
      tunnel: [w196] -> w162 mode=indexing
      i -> [w209]
      n67 = Multiply(x=w210, y=w209) -> (x*y=w207:i32)
      n68 = Add(x=w207, y=w208) -> (x+y=w206:i32)
